vi "Configure Output Enable Core.vi"(8 "error in (no error)":errorcluster, 9 "enabled (true)":bool=TRUE, 10 "channel name (\"CHANNEL1\")":string="CHANNEL1", 11 "IVI_DCPwr in":refnum<class "IVI_DCPwr.lvclass">) -> (0 "error out":errorcluster, 3 "IVI_DCPwr out":refnum<class "IVI_DCPwr.lvclass">)   [LabVIEW 2016, in "IVI_DCPwr.lvlib" / "IVI_DCPwr.lvclass"]
doc: "Configures whether the signal that the power supply produces on a channel appears at the output connector."
uses:
  IVI_DCPwr.lvclass
  IVI_DCPwr.lvclass/IVI_DCPwr.ctl
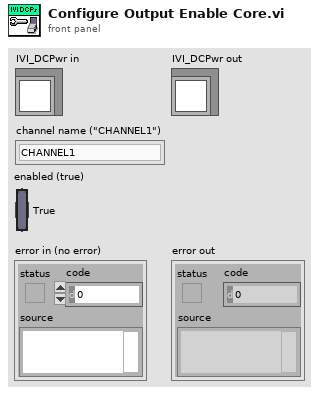
[diagram p1: front panel]
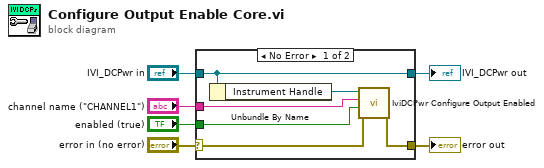
[diagram p0: block diagram]
diagram:
  n1 = case shown="No Error" "error in (no error)" {
    selector: "error in (no error)" -> [w10 w14]
    tunnel: [w9 w14] -> w5
    tunnel: [w12 w13] -> w3
    tunnel: "IVI_DCPwr in" -> [w12 w13]
    tunnel: "channel name (\"CHANNEL1\")" -> [w8 _]
    tunnel: "enabled (true)" -> [w7 _]
    frame No Error {
      n2 = Unbundle By Name(w12) -> ("Instrument Handle"=w11:refnum<k15>)
      n3 = call <vilib>:"IviDCPwr Configure Output Enabled.vi"("error in (no error)"=w10, "enabled (true)"=w7, "channel name (\"CHANNEL1\")"=w8, "instrument handle"=w11) -> ("error out"=w9:errorcluster)  [unwired: 6 in, 1 out]
    }
    frame Error {
    }
  }
  "error out" <- w5
  "IVI_DCPwr out" <- w3
